vi "build_xwav_from_units.vi"(0 "Y":dbl[](array[numeric]), 2 "units and scaling":T1={"y scaling factor (1)"=1.0, "scaled y units (au)"="counts", "x scaling factor / scaled dx (1)"=1.0, "x units (index)"="index", "scaled x0 (0)"=0.0, "x dimention (x)"="x"}, 3 "attributes":variant) -> (5 "xwave":T2={"attributes"=variant, "X"={"start"=1.0, "delta"=1.0, "units"="index", "dim"="au"}, "Y"={"data"=[], "units"="au"}})   [LabVIEW 2015]
uses:
  xwav.ctl
  xwav_units_and_scaling.ctl
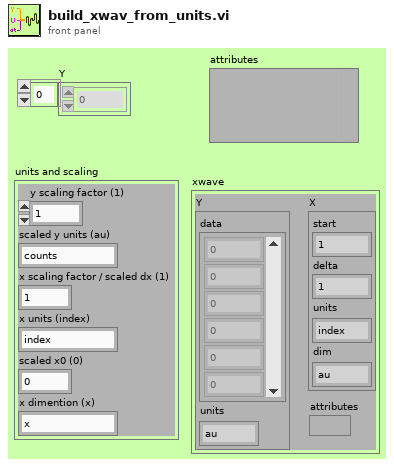
[diagram p1: front panel]
types:
  T1 = typedef "xwav_units_and_scaling.ctl" = cluster{"y scaling factor (1)":dbl, "scaled y units (au)":string, "x scaling factor / scaled dx (1)":dbl, "x units (index)":string, "scaled x0 (0)":dbl, "x dimention (x)":string}
  T2 = typedef "xwav.ctl" = cluster{"attributes":variant, "X":cluster{"start":dbl, "delta":dbl, "units":string, "dim":string}, "Y":cluster{"data":dbl[], "units":string}}
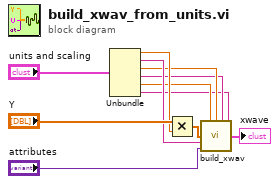
[diagram p0: block diagram]
diagram:
  n1 = Unbundle("units and scaling") -> ("y scaling factor (1)"=w6:dbl, "scaled y units (au)"=w5:string, "x scaling factor / scaled dx (1)"=w4:dbl, "x units (index)"=w3:string, "scaled x0 (0)"=w2:dbl, "x dimention (x)"=w1:string)
  n2 = Multiply(x="Y", y=w6) -> (x*y=w8:dbl[])
  n3 = call "build_xwav.vi"("x0 (0)"=w2, "dx (1)"=w4, "x units (index)"=w3, "x dimention (x)"=w1, "Y"=w8, "y units (au)"=w5, "attributes"="attributes") -> ("xwave"=→"xwave":T2)  [unwired: 8 in]
